vi "Test 2 Get Type Thee of a Kind.vi"(8 "error in (no error)":errorcluster, 11 "Test Case In":refnum<class "Day 7 Test.lvclass">) -> (0 "error out":errorcluster, 3 "Test Case Out":refnum<class "Day 7 Test.lvclass">)   [LabVIEW 2020, in "Day 7 Test.lvclass"]
uses:
  Day 7 Test.lvclass
  Day 7 Test.lvclass/Day 7 Test.ctl
  Hand/Hand.lvclass
  ffb4b03f-324e-4da4-84c3-4c0cc3f10137.vi
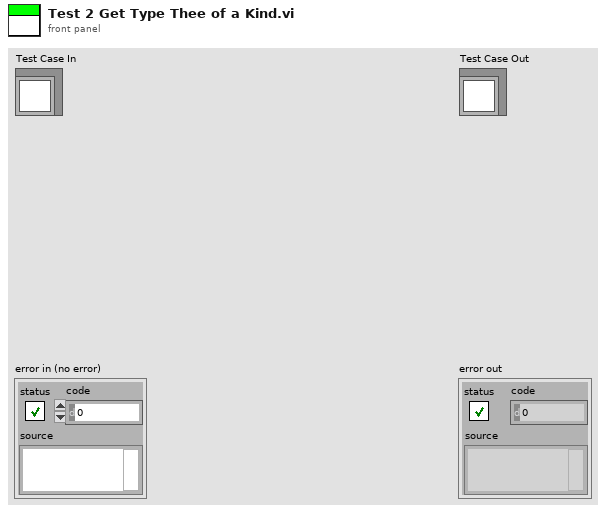
[diagram p1: front panel]
types:
  T1 = enum16{"High Card", "One Pair", "Two Pairs", "Three of a Kind", "Full House", "Four of a Kind", "Five of a Kind"}
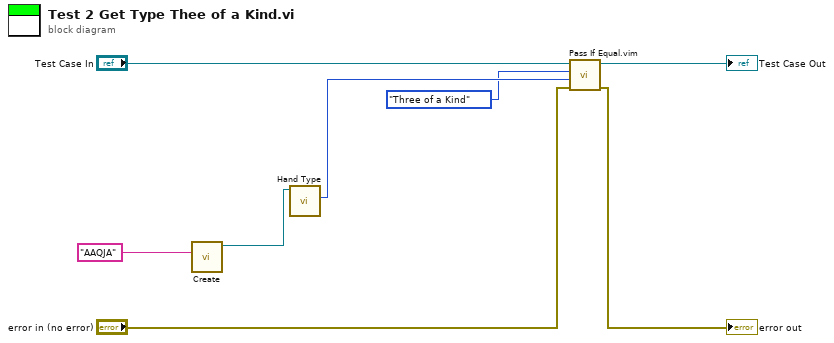
[diagram p0: block diagram]
diagram:
  n1 = call "Create.vi"("Input"="AAQJA") -> ("Hand"=w3:refnum<class "Hand.lvclass">)  [unwired: 9 in, 1 out]
  n2 = call "Hand Type.vi"("Hand In"=w3) -> ("Score"=w2:T1)  [unwired: 8 in, 2 out]
  n3 = call "Pass If Equal.vim"("error in (no error)"="error in (no error)", "Actual"=w2, "Expected"=T1."Three of a Kind" ("Score"), "LUnit Test Case In"="Test Case In") -> ("error out"=→"error out":errorcluster, "LUnit Test Case Out"=→"Test Case Out":refnum<class "Day 7 Test.lvclass">)  [unwired: 6 in]
